vi "LV FPGA Serial Read Write v2.vi"() -> ()   [LabVIEW 2014]
uses:
  <vilib>/rvi/Emulation/niFpgaGetClockAttributes.vi
  <vilib>/rvi/Emulation/niFpgaSctlEmulationGetInTimedLoop.vi
  <vilib>/rvi/Emulation/niFpgaEmulationReportErrorSimple.vi
  Controls/Stop.vi
  <vilib>/rvi/eio/common/nirviEmuTemplateMethod_errors.vi
  <vilib>/rvi/Emulation/niFpgaCriticalErrorInLSC.vi
  <vilib>/rvi/Emulation/niFpgaEmulationIsFPGAContextNoSignature.vi
  <vilib>/rvi/errors/niFpgaSetErrorForExecOnDevCompSimple.vi
  <vilib>/rvi/eio/common/nirviEmuReportErrorAndStop.vi
  <vilib>/rvi/DataTransferAndStorage/Container/Common/niFpgaContainerGetUniqueNameForEmu.vi
  <vilib>/rvi/FIFO/Fifo_Resource/nirvififoEmulationSetSize.vi
  <vilib>/rvi/FIFO/Fifo_Resource/nirviFifoEmulationQueueMgr.vi
  <instcachedir>/0/nirviFifoEmulationQueueMgr_E5CAEC123FF24DC58D834DCA3CDAA9B5.lvgen/nirviFifoEmulationQueueMgr_E5CAEC123FF24DC58D834DCA3CDAA9B5_000.vi
  <vilib>/rvi/FIFO/Fifo_Resource/nirvififoEmulationDetermineInputValidOut.vi
  <vilib>/rvi/FIFO/Fifo_Resource/nirvififoEmulationCreateLock.vi
  <vilib>/rvi/Emulation/niFpgaProcessEmulError.vi
  <vilib>/rvi/FIFO/Fifo_Resource/nirvififoEmulationObtainLock.vi
  <vilib>/rvi/FIFO/Fifo_Resource/nirvififoEmulationReleaseLock.vi
  <vilib>/rvi/occurrence/nirviWaitOnOccurrenceBase.vi
  <vilib>/rvi/errors/nirviReportUnexpectedCaseInternalError.vi
  <vilib>/rvi/errors/nirviReportUnexpectedCaseInternalError (U32).vi
  <vilib>/eio/EIONode/EIONode.xnode
  <vilib>/rvi/DataTransferAndStorage/Container/XNode/niFpgaContainer.xnode
  <vilib>/rvi/FIFO/Fifo_Resource/nirvififoEmulationWrite.vi
panel:
  out "Read: Transmission Error":bool
  in  "Invert Polarity?":bool
  in  "parity (0:none)":enum16{"None", "Odd", "Even", "Mark", "Space"}(ring)
  in  "data bits (8)":i32=8 min=5 max=8 step=1
  in  "Receive":refnum<k21>="ConnectorA/DIO10"
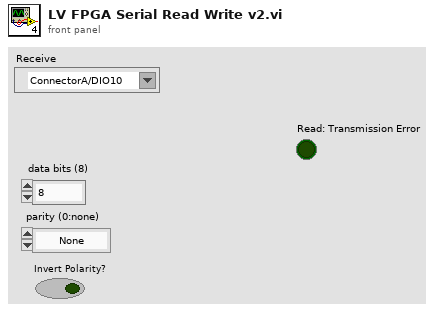
[diagram p1: front panel]
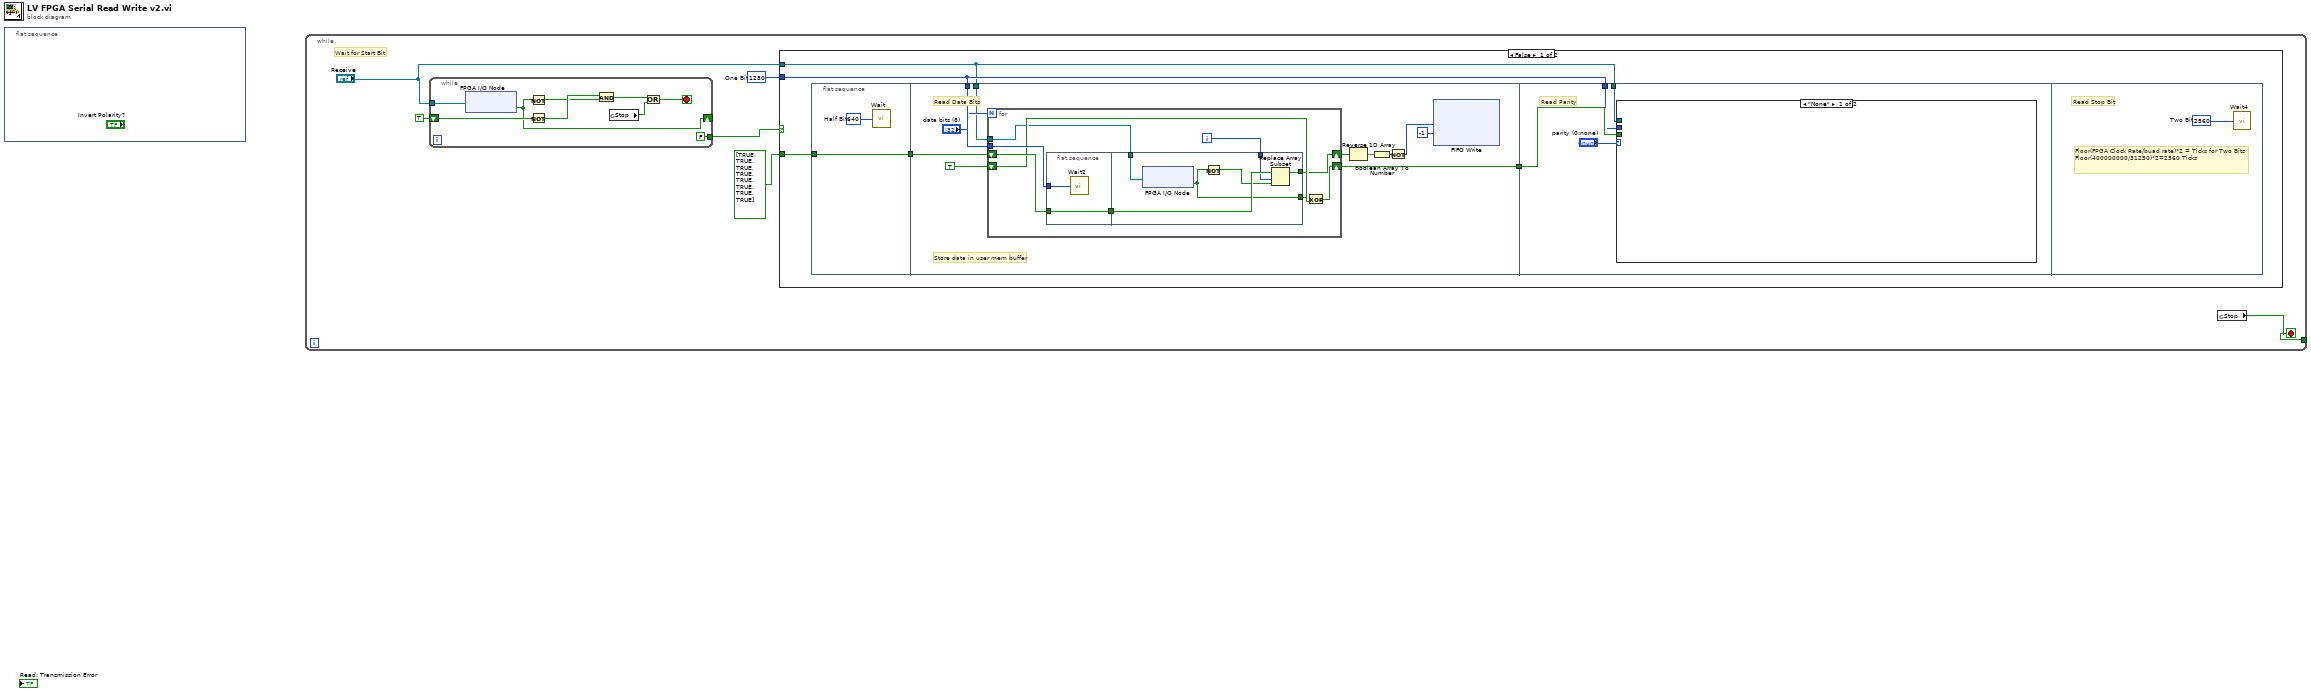
[diagram p0: block diagram]
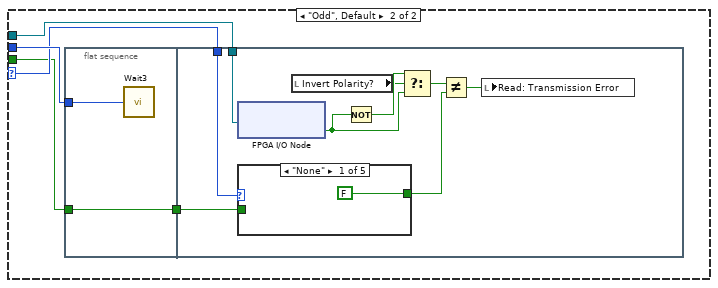
[diagram p2: hidden frame]
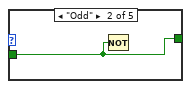
[diagram p3: hidden frame]
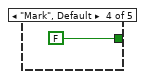
[diagram p5: hidden frame]
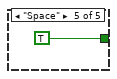
[diagram p6: hidden frame]
diagram:
  n1 = flat-sequence {
    frame #0 {
    }
  }
  n2 = while {
    tunnel: [w2] -> _
    stop <- w2 stop-if-true
    w1 = u32 1280  # One Bit
    # "Wait for Start Bit"
    n3 = while {
      tunnel: [FALSE] -> w5
      shift-right: [w7] -> _
      shift-left: TRUE -> [w14]
      tunnel: "Receive" -> [w10]
      stop <- w11 stop-if-true
      n4 = xnode "FPGA I/O Node"("FPGA I/O In"=w10) -> ("I/O Item"=w7:bool)  [unwired: 1 out]
      n5 = Not(x=w7) -> (.not. x?=w8:bool)
      n6 = Not(x=w14) -> (.not. x?=w13:bool)
      n7 = And(x=w13, y=w8) -> (x .and. y?=w12:bool)
      n8 = global read "Stop.vi" "Stop"() -> (w9:bool)
      n9 = Or(x=w12, y=w9) -> (x .or. y?=w11:bool)
    }
    n10 = case shown="False" w5 {
      tunnel: bool[] [TRUE, TRUE, TRUE, TRUE, TRUE, TRUE, TRUE, TRUE] -> [w19 _]
      tunnel: w1 -> [w18 _]
      tunnel: "Receive" -> [w16 _]
      frame False {
        n11 = flat-sequence {
          tunnel: [w22] -> w20
          tunnel: w19 -> [w22]
          tunnel: w20 -> [w33]
          tunnel: w18 -> [w32]
          tunnel: [w30] -> w17
          tunnel: w16 -> [w28]
          tunnel: w18 -> [w52]
          tunnel: w17 -> [w54]
          tunnel: w16 -> [w51]
          frame #0 {
            w21 = u32 640  # Half Bit
            n12 = call "Wait"("Count(Ticks)"=w21) -> ()  [unwired: 1 out]
          }
          frame #1 {
            # "Store data in user mem buffer"
            # "Read Data Bits"
            n13 = for {
              N: "data bits (8)" -> [_]
              shift-right: [w36] -> w26
              shift-left: w33 -> [w42]
              tunnel: w32 -> [w40]
              shift-right: [w39] -> w30
              shift-left: TRUE -> [w38]
              tunnel: w28 -> [w35]
              i -> [w34]
              n14 = flat-sequence {
                tunnel: w42 -> [w44]
                tunnel: [w44] -> w41
                tunnel: w40 -> [w43]
                tunnel: w41 -> [w50]
                tunnel: [w49] -> w36
                tunnel: [w47] -> w37
                tunnel: w35 -> [w48]
                tunnel: w34 -> [w46]
                frame #0 {
                  n15 = call "Wait2"("Count(Ticks)"=w43) -> ()  [unwired: 1 out]
                }
                frame #1 {
                  n16 = xnode "FPGA I/O Node"("FPGA I/O In"=w48) -> ("I/O Item"=w47:bool)  [unwired: 1 out]
                  n17 = Not(x=w47) -> (.not. x?=w45:bool)
                  n18 = Replace Array Subset(array=w50, new element=w45, index=w46) -> (w49:bool[])
                }
              }
              n19 = Exclusive Or(1:w38, 2:w37) -> (0:w39:bool)
            }
            n20 = Reverse 1D Array(array=w26) -> (reversed array=w25:bool[])
            n21 = Boolean Array To Number(Boolean array=w25) -> (number=w24:u8)
            n22 = Not(x=w24) -> (.not. x?=w23:u8)
            n23 = xnode ("FIFO Write")("Element"=w23, "Timeout"=-1) -> ()  [unwired: 1 in, 2 out]
          }
          frame #2 {
            # "Read Parity"
            n24 = case shown="\"None\"" "parity (0:none)" {
              selector: "parity (0:none)" -> [_ w58]
              tunnel: w54 -> [_ w56]
              tunnel: w52 -> [_ w59]
              tunnel: w51 -> [_ w55]
              frame "None" {
              }
              frame "Odd", Default {
                n25 = flat-sequence {
                  tunnel: w59 -> [w61]
                  tunnel: [w60] -> w57
                  tunnel: w56 -> [w60]
                  tunnel: w58 -> [w70]
                  tunnel: w57 -> [w68]
                  tunnel: w55 -> [w66]
                  frame #0 {
                    n26 = call "Wait3"("Count(Ticks)"=w61) -> ()  [unwired: 1 out]
                  }
                  frame #1 {
                    n27 = xnode "FPGA I/O Node"("FPGA I/O In"=w66) -> ("I/O Item"=w63:bool)  [unwired: 1 out]
                    n28 = case shown="\"None\"" w70 {
                      tunnel: w68 -> [_ w72 w73 _ _]
                      tunnel: [FALSE ("y") w72 w73 FALSE ("y") TRUE ("y")] -> w69
                      frame "None" {
                      }
                      frame "Odd" {
                        n29 = Not(x=w72) -> ()  [unwired: 1 out]
                      }
                      frame "Even" {
                      }
                      frame "Mark", Default {
                      }
                      frame "Space" {
                      }
                    }
                    n30 = local read "Invert Polarity?"() -> (w64:bool)
                    n31 = Not(x=w63) -> (.not. x?=w65:bool)
                    n32 = Select(t=w65, s=w64, f=w63) -> (s? t:f=w62:bool)
                    n33 = Not Equal?(x=w62, y=w69) -> (x != y?=w67:bool)
                    n34 = local write "Read: Transmission Error"(w67) -> ()
                  }
                }
              }
            }
          }
          frame #3 {
            w76 = u32 2560  # Two Bit
            # "Floor(FPGA Clock Rate/buad rate)*2 = Ticks for Two Bits\nFloor(400000000/31250)*2=2560 Ticks"
            # "Read Stop Bit"
            n35 = call "Wait4"("Count(Ticks)"=w76) -> ()  [unwired: 1 out]
          }
        }
      }
      frame True {
      }
    }
    n36 = global read "Stop.vi" "Stop"() -> (w2:bool)
  }
